vi "Arrange VIWin - Compute Window Bounds.vi"(0 "display workspace bounds":T1, 1 "content rectangle":T5, 5 "window bounds":T2, 7 "min window dimensions":T3, 9 "window gaps":T4) -> (4 "window bounds":T1)   [LabVIEW 2020, in "Arrange VI Window.lvlib"]
uses:
  Arrange VI Window.lvlib
  Arrange VIWin - Rectangle Dimensions.ctl
  Arrange VIWin - Window Gaps.ctl
  Arrange VIWin - Min Window Dimensions.ctl
  Arrange VIWin - Window Margins.ctl
  <vilib>/Utility/miscctls.llb/LVRectTypeDef.ctl
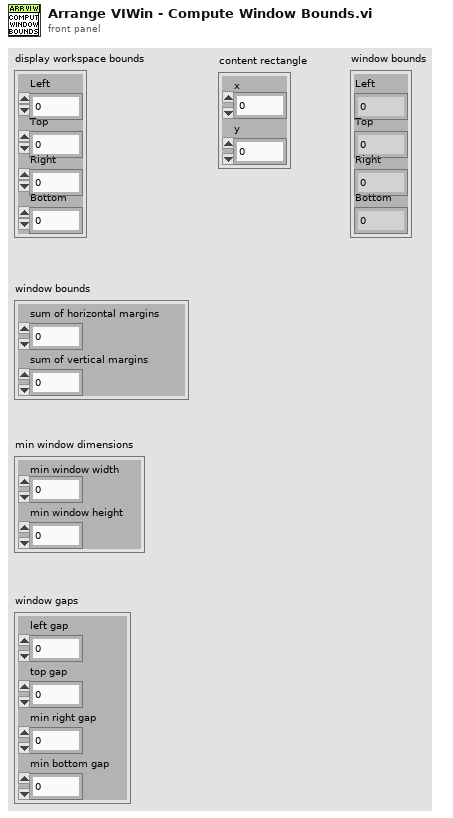
[diagram p1: front panel]
types:
  T1 = typedef "LVRectTypeDef.ctl" = cluster{"Left":i16, "Top":i16, "Right":i16, "Bottom":i16}
  T2 = typedef "Arrange VI Window.lvlib/Arrange VIWin - Window Margins.ctl" = cluster{"sum of horizontal margins":i16, "sum of vertical margins":i16}
  T3 = typedef "Arrange VI Window.lvlib/Arrange VIWin - Min Window Dimensions.ctl" = cluster{"min window width":i16, "min window height":i16}
  T4 = typedef "Arrange VI Window.lvlib/Arrange VIWin - Window Gaps.ctl" = cluster{"left gap":i16, "top gap":i16, "min right gap":i16, "min bottom gap":i16}
  T5 = typedef "Arrange VI Window.lvlib/Arrange VIWin - Rectangle Dimensions.ctl" = cluster{"x":i16, "y":i16}
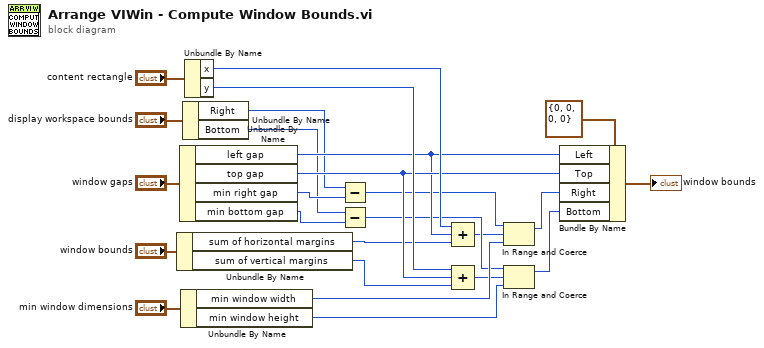
[diagram p0: block diagram]
diagram:
  n1 = Unbundle By Name("window bounds") -> ("sum of horizontal margins"=w14:i16, "sum of vertical margins"=w15:i16)
  n2 = Unbundle By Name("window gaps") -> ("left gap"=w19:i16, "top gap"=w22:i16, "min right gap"=w21:i16, "min bottom gap"=w20:i16)
  n3 = Unbundle By Name("min window dimensions") -> ("min window width"=w16:i16, "min window height"=w17:i16)
  n4 = Unbundle By Name("display workspace bounds") -> ("Right"=w5:i16, "Bottom"=w6:i16)
  n5 = Unbundle By Name("content rectangle") -> ("x"=w25:i16, "y"=w24:i16)
  n6 = Subtract(x=w5, y=w21) -> (x-y=w7:i16)
  n7 = Subtract(x=w6, y=w20) -> (x-y=w8:i16)
  n8 = Compound Arithmetic op=ADD(w25, w19, w14) -> (w3:i16)
  n9 = Compound Arithmetic op=ADD(w24, w22, w15) -> (w2:i16)
  n10 = In Range and Coerce(upper limit=w7, x=w3, lower limit=w16) -> (coerced(x)=w10:i16)  [unwired: 1 out]
  n11 = In Range and Coerce(upper limit=w8, x=w2, lower limit=w17) -> (coerced(x)=w4:i16)  [unwired: 1 out]
  n12 = Bundle By Name(cluster=T1 {"Left"=0, "Top"=0, "Right"=0, "Bottom"=0} ("Block Diagram Window:Window Bounds"), "Left"=w19, "Top"=w22, "Right"=w10, "Bottom"=w4) -> (→"window bounds":T1)
